vi "8 and 4 pulses TX 8spc.vi"(7 "reset system clock":bool, 8 "referenses":T1={"clock x2"="IO Socket\\Data Clock 2x", "Memory In"="pulse on memory", "Memory In 2"="pulse on memory", "Memory In 3"="pulse on memory", "Memory In 4"="pulse on memory"}, 9 "IQ_run":bool=TRUE, 10 "PDW input Valid":bool, 11 "array PDW":u64[](array[numeric])=[0, 0, 0, 0]) -> (0 "trig out":bool, 1 "pulse TX status":T2, 2 "output valid":bool, 3 "IQ out":T3[](array[typedef]), 4 "ready for input":bool)   [LabVIEW 2021]
uses:
  <instrlib>/_niInstr/DSP/v1/Shared/Public/IQ Data.ctl
  pulse_tx_vis/CTL/mode_type.ctl
  <instrlib>/_niInstr/Basic Elements/v1/FPGA/Private/Count Up U64.vi
  <instrlib>/_niInstr/Basic Elements/v1/FPGA/Private/Count Up U32.vi
  <instrlib>/_niInstr/Basic Elements/v1/FPGA/niInstr Basic Elements v1 FPGA.lvlib
  <instrlib>/_niInstr/DSP/v1/Shared/niInstr DSP v1 Shared.lvlib
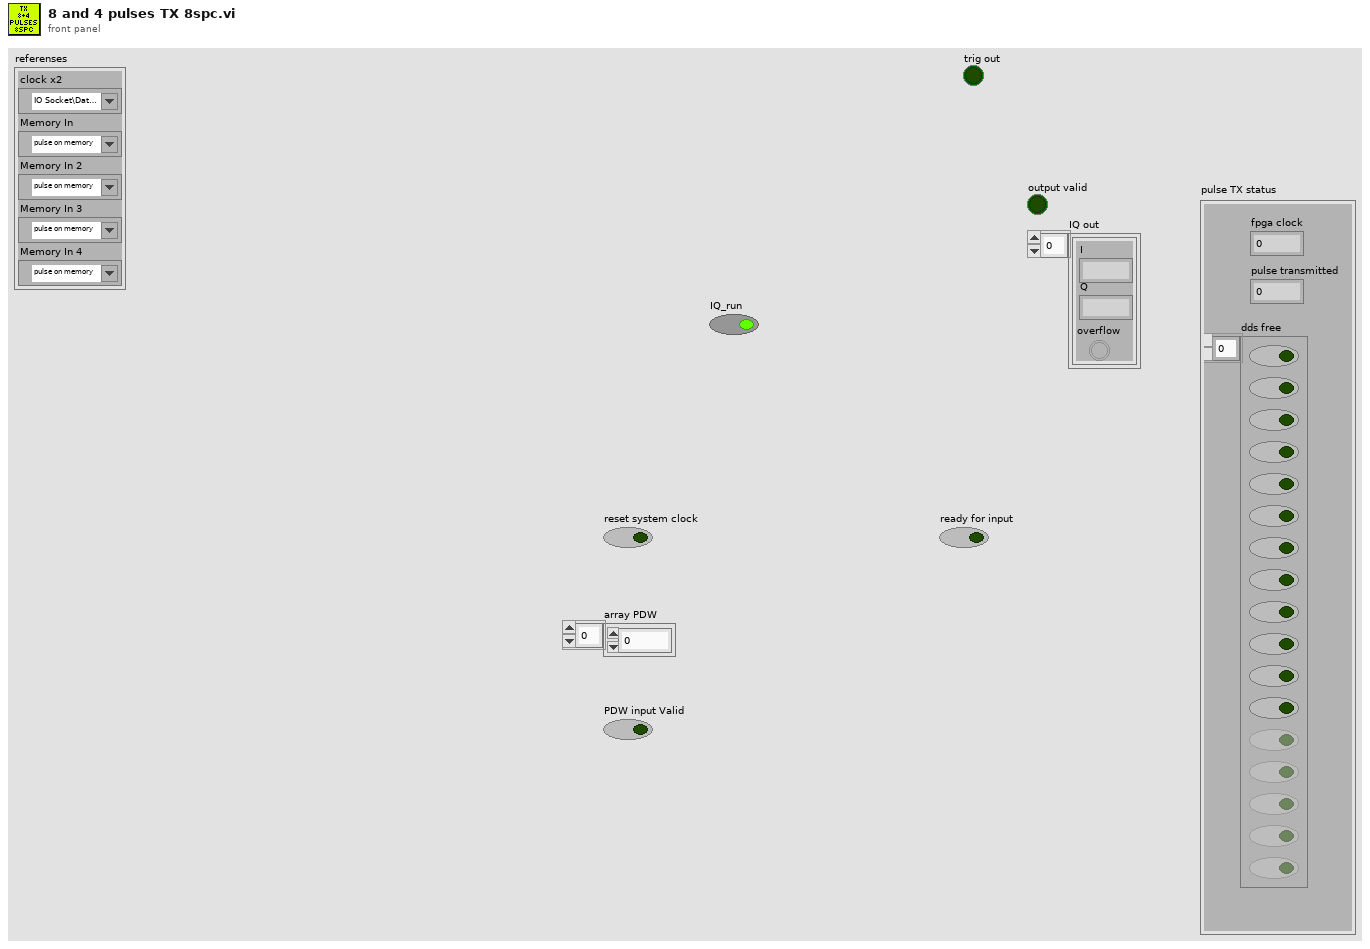
[diagram p1: front panel]
types:
  T1 = cluster{"clock x2":refnum<k21>, "Memory In":refnum<k21>, "Memory In 2":refnum<k21>, "Memory In 3":refnum<k21>, "Memory In 4":refnum<k21>}
  T2 = cluster{"fpga clock":u64, "pulse transmitted":u32, "dds free":bool[]}
  T3 = typedef "niInstr DSP v1 Shared.lvlib/IQ Data.ctl" = cluster{"I":fxp<+/-,18,1>, "Q":fxp<+/-,18,1>, "overflow":bool}
  T4 = typedef "mode_type.ctl" = enum8{"CW", "from memory 1", "NC - cw", "LFM", "BPSK", "QPSK"}
  T5 = typedef "pdw.ctl" = cluster{"PW":u32, "frequency shift":fxp<+/-,48,0>, "amp":fxp<+/-,18,1>, "mode type":T4, "mode depth":u32, "mode filter":u8, "phase shift":fxp<+/-,16,1>, "pulse shape filter":u8}
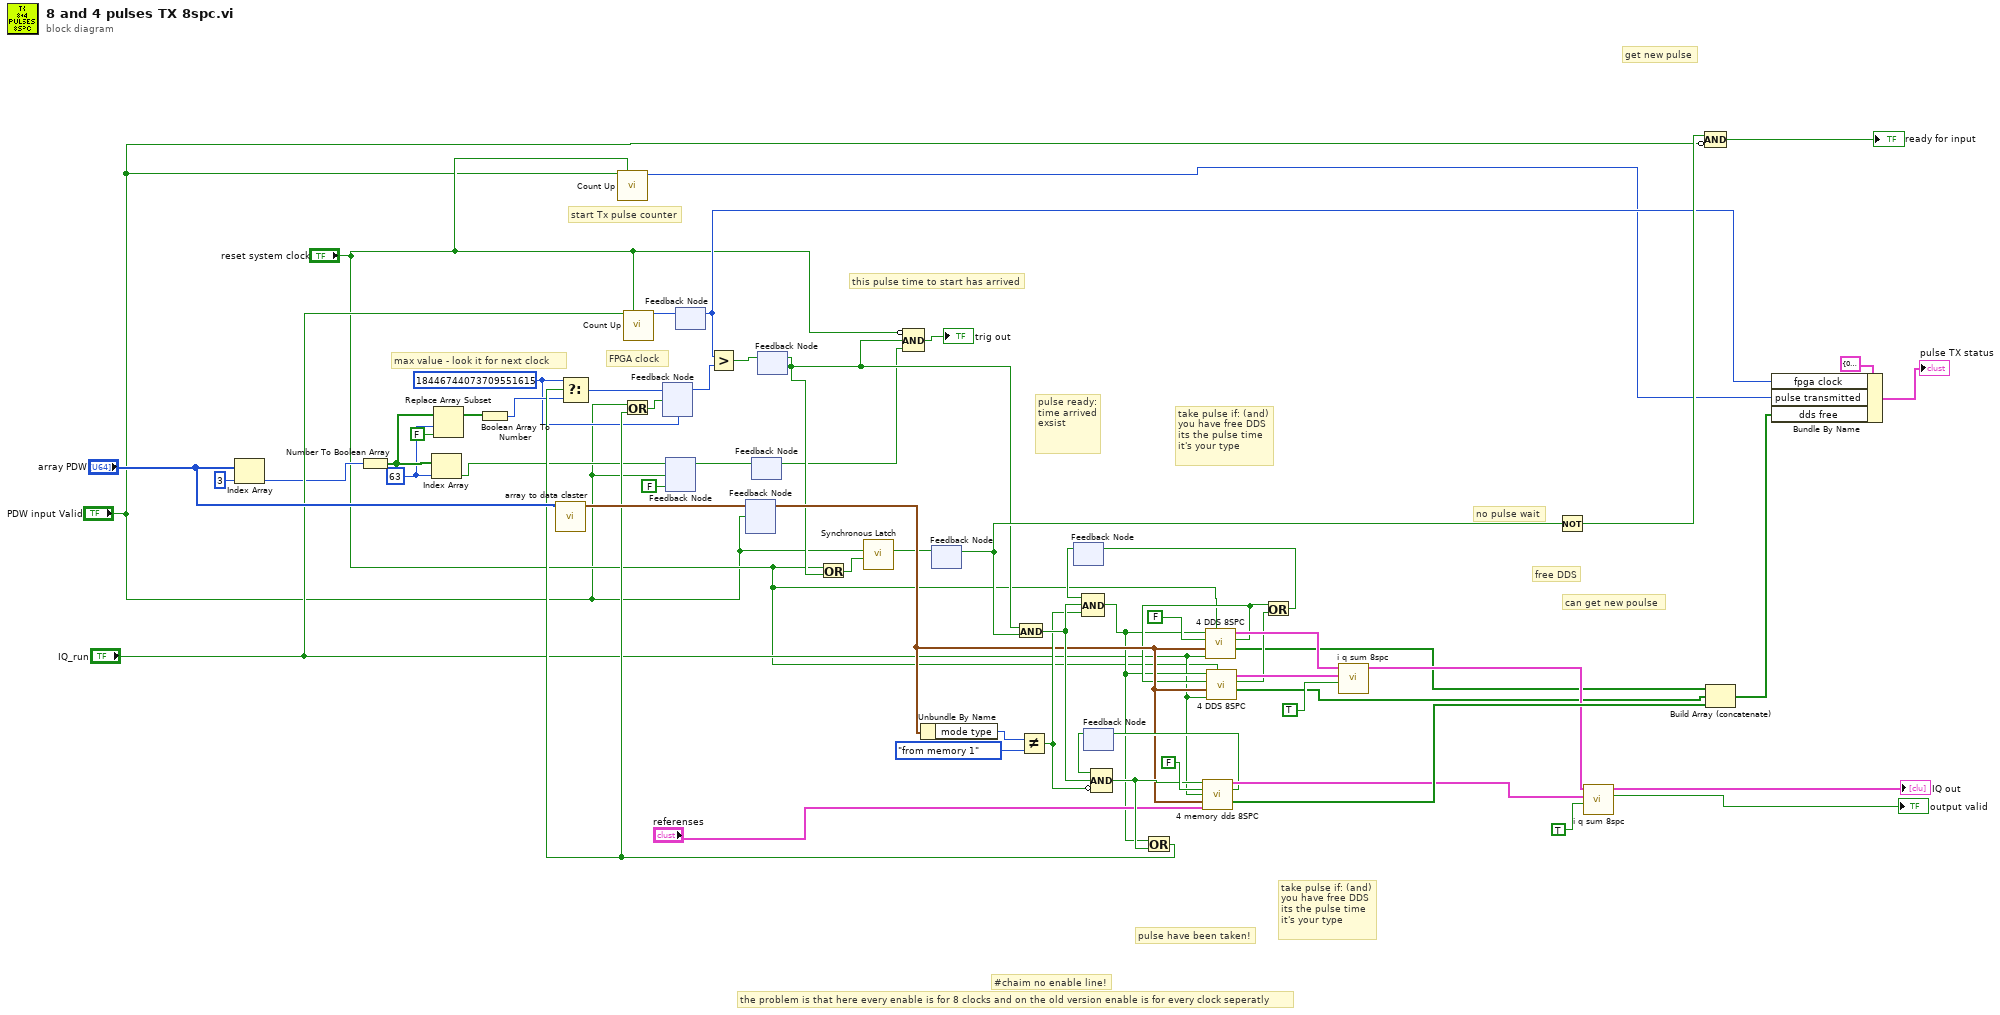
[diagram p0: block diagram]
diagram:
  w15 = 63 ("index")
  w5 = u64 18446744073709551615 ("t")
  # "pulse ready:\ntime arrived\nexsist"
  # "take pulse if: (and)\nyou have free DDS\nits the pulse time\nit's your type"
  # "take pulse if: (and)\nyou have free DDS\nits the pulse time\nit's your type"
  # "pulse have been taken!"
  # "the problem is that here every enable is for 8 clocks and on the old version enable is for every clock seperatly"
  # "#chaim no enable line!"
  # "start Tx pulse counter"
  # "FPGA clock"
  # "this pulse time to start has arrived"
  # "max value - look it for next clock"
  # "get new pulse"
  # "can get new poulse"
  # "no pulse wait"
  # "free DDS"
  n1 = Index Array(array="array PDW", index=3) -> (element=w12:u64)
  n2 = Number To Boolean Array(number=w12) -> (Boolean array=w16:bool[])
  n3 = Index Array(array=w16, index=w15) -> (element=w10:bool)
  n4 = Replace Array Subset(array=w16, new element=FALSE ("new element/subarray"), index=w15) -> (w13:bool[])
  n5 = Boolean Array To Number(Boolean array=w13) -> (number=w11:u64)
  n6 = call "array to data claster.vi"("Array"="array PDW") -> ("Cluster"=w46:T5)  [unwired: 10 in]
  n7 = call-poly <instrlib>:"Count Up.vi"("increment"="PDW input Valid", "reset"="reset system clock") -> ("count out"=w50:u32)  [unwired: 13 in]
  n8 = call-poly <instrlib>:"Count Up.vi"("increment"="IQ_run", "reset"="reset system clock") -> ("count out"=w58:u64)  [unwired: 13 in]
  n9 = feedback #1(w5) -> (w54:u64)
  n10 = feedback #2(FALSE) -> (w2:bool)
  n11 = feedback-in #2(w10, "PDW input Valid") -> ()
  n12 = feedback #3() -> (w51:u64)  [unwired: 1 in]
  n13 = feedback-in #3(w58) -> ()
  n14 = Greater?(x=w51, y=w54) -> (0:w62:bool)
  n15 = feedback #4() -> (w31:T5)  [unwired: 1 in]
  n16 = feedback-in #4(w46, "PDW input Valid") -> ()
  n17 = feedback #5() -> (w1:bool)  [unwired: 1 in]
  n18 = feedback-in #5(w2) -> ()
  n19 = feedback #6() -> (w8:bool)  [unwired: 1 in]
  n20 = feedback-in #6(w62) -> ()
  n21 = Or(x="reset system clock", y=w8) -> (x .or. y?=w20:bool)
  n22 = call <instrlib>:"Synchronous Latch.vi"("clear"=w20, "set"="PDW input Valid") -> ("out"=w18:bool)  [unwired: 9 in]
  n23 = Compound Arithmetic op=AND(invert "reset system clock", w8, w1) -> (→"trig out":bool)
  n24 = Unbundle By Name(w31) -> ("mode type"=w48:T4)
  n25 = feedback #7() -> (w17:bool)  [unwired: 1 in]
  n26 = feedback-in #7(w18) -> ()
  n27 = And(x=w8, y=w17) -> (x .and. y?=w43:bool)
  n28 = Not Equal?(x=w48, y=mode_type."from memory 1") -> (x != y?=w42:bool)
  n29 = feedback #8() -> (w32:bool)  [unwired: 1 in]
  n30 = Compound Arithmetic op=AND(w32, w43, w42) -> (w23:bool)
  n31 = feedback #9() -> (w36:bool)  [unwired: 1 in]
  n32 = Compound Arithmetic op=AND(w36, w43, invert w42) -> (w35:bool)
  n33 = Or(x=w23, y=w35) -> (x .or. y?=w34:bool)
  n34 = Select(t=w5, s=w34, f=w11) -> (s? t:f=w57:u64)
  n35 = Or(x="PDW input Valid", y=w34) -> (x .or. y?=w9:bool)
  n36 = feedback-in #1(w57, w9) -> ()
  n37 = call "4 memory dds 8SPC.vi"("new PDW in"=w35, "free DDS before me?"=FALSE, "run"="IQ_run", "pdw in"=w31, "referenses"="referenses") -> ("IQ out"=w38:T3[], "have free DDS"=w37:bool, "state of every DDS"=w40:bool[])  [unwired: 7 in, 1 out]
  n38 = feedback-in #9(w37) -> ()
  n39 = call "4 DDS 8SPC.vi"("clear DDS"="reset system clock", "input valid"="IQ_run", "pdw in"=w31, "free DDS before me?"=FALSE, "new PDW in"=w23) -> ("state of every DDS"=w22:bool[], "have free DDS"=w24:bool, "IQ out"=w30:T3[])  [unwired: 3 in, 1 out]
  n40 = call "4 DDS 8SPC.vi"("clear DDS"="reset system clock", "input valid"="IQ_run", "pdw in"=w31, "free DDS before me?"=w24, "new PDW in"=w23) -> ("state of every DDS"=w21:bool[], "have free DDS"=w26:bool, "IQ out"=w29:T3[])  [unwired: 3 in, 1 out]
  n41 = Or(x=w24, y=w26) -> (x .or. y?=w25:bool)
  n42 = feedback-in #8(w25) -> ()
  n43 = call "i q sum 8spc.vi"("input valid"=TRUE, "IQ in 2"=w29, "IQ in"=w30) -> ("IQ out"=w28:T3[])  [unwired: 7 in, 1 out]
  n44 = Not(x=w17) -> (.not. x?=w55:bool)
  n45 = call "i q sum 8spc.vi"("input valid"=TRUE, "IQ in 2"=w38, "IQ in"=w28) -> ("output valid"=→"output valid":bool, "IQ out"=→"IQ out":T3[])  [unwired: 7 in]
  n46 = Compound Arithmetic op=AND(w55, invert "PDW input Valid") -> (→"ready for input":bool)
  n47 = Build Array (concatenate)(w22, w21, w40) -> (w49:bool[])
  n48 = Bundle By Name(cluster=T2 {"fpga clock"=0, "pulse transmitted"=0, "dds free"=[FALSE, FALSE, FALSE, FALSE, FALSE, FALSE, FALSE, FALSE, FALSE, FALSE, FALSE, FALSE]} ("pulse TX status"), "fpga clock"=w51, "pulse transmitted"=w50, "dds free"=w49) -> (→"pulse TX status":T2)
